vi "Periodic Tasks.vi"(8 "error in":errorcluster) -> ()   [LabVIEW 2017]
doc: "This VI runs in parallel to other tasks. It can contain as many user-defined periodic loops as you need. These can carry out PID or other sorts of timed response."
uses:
  <vilib>/Rock Robotics/WPI/DriverStation/WPI_DriverStationRobotMode2.ctl
  <vilib>/Rock Robotics/WPI/Utilities/WPI_GetSetVariantRefNum.vi
  Robot Global Data.vi
  <vilib>/Rock Robotics/Network Tables/NT Write Number.vi
  <vilib>/Rock Robotics/WPI/ThirdParty/Sensors/ADIS16448 IMU/ADIS16448_IMU.lvlib
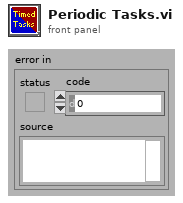
[diagram p1: front panel]
types:
  T1 = typedef "WPI_PotentiometerDevRef.ctl" = cluster{"DevStatus":errorcluster, "Analog Channel":T2, "Invert Output":bool}
  T2 = typedef "FPGA_AIChannel.ctl" = enum8{"AI 0", "AI 1", "AI 2", "AI 3", "AI MXP 0", "AI MXP 1", "AI MXP 2", "AI MXP 3", "Invalid"}
  T3 = typedef "ADIS16448_IMU.lvlib/ADI_IMU_ADIS16448_IMUDevRef.ctl" = cluster{"DevStatus":errorcluster, "Handle":i32, "SPI Bus":T4, "Device Found":bool, "Device Ready":bool, "Yaw Axis":enum16{"X", "Y", "Z"}, "AHRS Algorithm":enum16{"Complementary", "Madgwick"}, "Serial":u16, "Lot ID 2":u16, "Lot ID 1":u16, "Bytes Per Sample":u16, "Calibrate On Open?":bool}
  T4 = typedef "spi_bus.ctl" = enum16{"SPI On-Board, CS0", "SPI On-Board, CS1", "SPI On-Board, CS2", "SPI On-Board, CS3", "SPI MXP", "Invalid"}
  T5 = typedef "WPI_EncoderDevRef.ctl" = cluster{"DevStatus":errorcluster, "EncoderIndex":T6, "CounterIndex":T7, "DistancePerCount":dbl, "Decoding Type":T8}
  T6 = typedef "FPGA_EncoderIdx.ctl" = enum8{"Enc 0", "Enc 1", "Enc 2", "Enc 3", "Enc 4", "Enc 5", "Enc 6", "Enc 7", "Invalid"}
  T7 = typedef "FPGA_CounterCtrSystemIndex.ctl" = enum8{"Ctr 0", "Ctr 1", "Ctr 2", "Ctr 3", "Ctr 4", "Ctr 5", "Ctr 6", "Ctr 7", "Invalid"}
  T8 = typedef "WPI_EncoderType.ctl" = enum16{"1x", "2x", "4x"}
  T9 = typedef "WPI_JoystickDevRef.ctl" = cluster{"Device":T10}
  T10 = typedef "WPI_JoystickDeviceEnum.ctl" = enum16{"USB 0", "USB 1", "USB 2", "USB 3", "USB 4", "USB 5"}
  T11 = typedef "WPI_RobotDriveDevRef.ctl" = cluster{"DevStatus":errorcluster, "Motors[]":T12[], "Square Inputs":bool, "Max Output":dbl}
  T12 = typedef "WPI_MotorControlDeviceRef.ctl" = cluster{"DeviceStatus":errorcluster, "Type":T13, "PWM":cluster{"PWM Channel":T14, "DeadBand":T15}, "CAN":cluster{"Device Number":u8, "SetOutput VI Ref":variant, "GetOutput VI Ref":variant, "Enable VI Ref":variant, "Disable VI Ref":variant, "Data":variant}, "Invert":bool, "DIO PWM":cluster{"PWM \"Enable\" Channel":T14, "DIOChannel":T16, "PWM Rate":dbl}}
  T13 = typedef "WPI_MotorControlType.ctl" = enum16{"PWM", "CAN", "DIO PWM"}
  T14 = typedef "FPGA_DIOPWMChannel.ctl" = enum8{"PWM 0", "PWM 1", "PWM 2", "PWM 3", "PWM 4", "PWM 5", "PWM 6", "PWM 7", "PWM 8", "PWM 9", "PWM MXP 0", "PWM MXP 1", "PWM MXP 2", "PWM MXP 3", "PWM MXP 4", "PWM MXP 5", "PWM MXP 6", "PWM MXP 7", "PWM MXP 8", "PWM MXP 9", "Invalid"}
  T15 = typedef "WPI_PWMDeadband.ctl" = cluster{"Name":string, "maxPositivePwm":i32, "minPositivePwm":i32, "centerPwm":i32, "maxNegativePwm":i32, "minNegativePwm":i32, "angularRange":u16}
  T16 = typedef "FPGA_DIOChannel.ctl" = enum8{"DIO 0", "DIO 1", "DIO 2", "DIO 3", "DIO 4", "DIO 5", "DIO 6", "DIO 7", "DIO 8", "DIO 9", "DIO MXP 0", "DIO MXP 1", "DIO MXP 2", "DIO MXP 3", "DIO MXP 4", "DIO MXP 5", "DIO MXP 6", "DIO MXP 7", "DIO MXP 8", "DIO MXP 9", "DIO MXP 10", "DIO MXP 11", "DIO MXP 12", "DIO MXP 13", "DIO MXP 14", "DIO MXP 15", "SPI Port CS1", "SPI Port CS2", "SPI Port CS3", "SPI Port MISO", "SPI Port MOSI", "Invalid"}
  T17 = cluster{"JoystickDevRef":T9, "RobotDriveDevRef":T11, "PotDevRef":T1, "ADI IMU DevRef":T3, "EncoderDevRef":T5, "EncoderDevRef":T5}
  T18 = typedef "WPI_DriverStationRobotMode2.ctl" = enum16{"Autonomous Disabled", "Autonomous Enabled", "Teleop Disabled", "Teleop Enabled", "Disconnected", "Finish", "Test Disabled", "Test Enabled", "Emergency Stopped"}
  T19 = cluster{"X Angle":dbl, "Y Angle":dbl, "Z Angle":dbl}
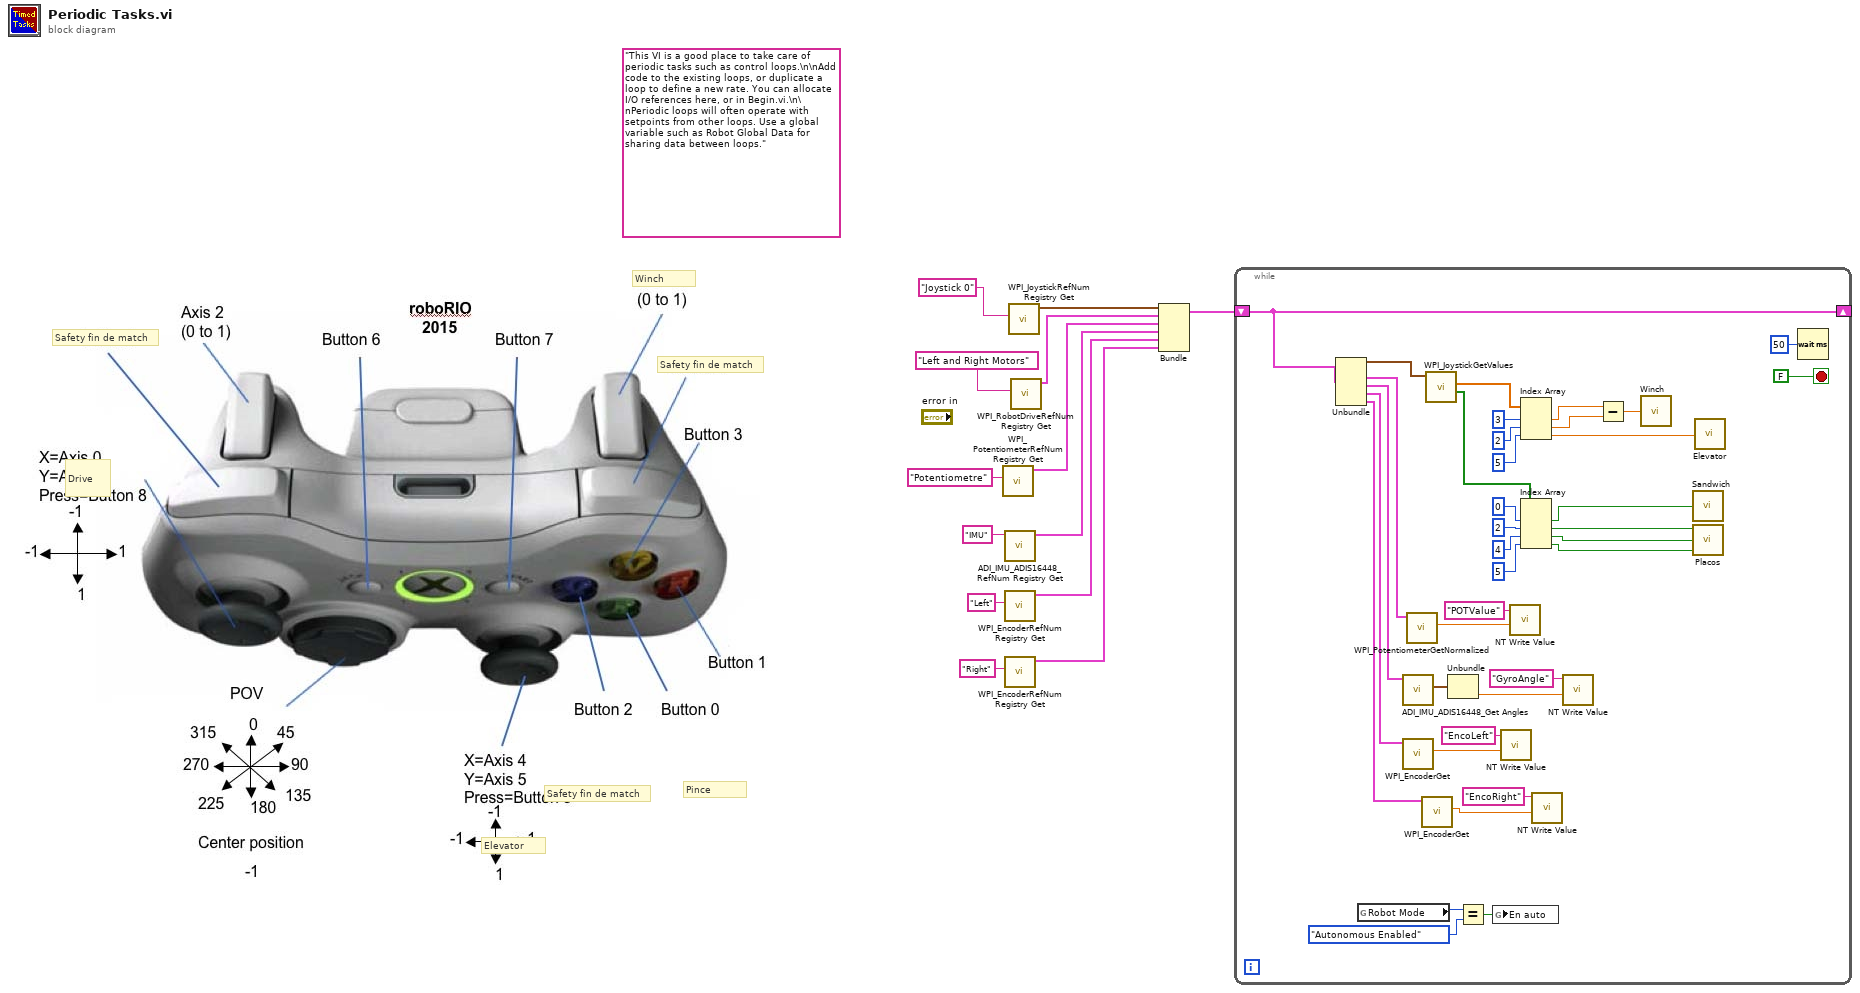
[diagram p0: block diagram]
diagram:
  (unwired) "This VI is a good place to take care of periodic tasks such as control loops.\n\nAdd code to the existing loops, or duplicate a loop to define a new rate. You can allocate I/O references here, or in Begin.vi.\n\nPeriodic loops will often operate with setpoints from other loops. Use a global variable such as Robot Global Data for sharing data between loops."
  # "Safety fin de match"
  # "Safety fin de match"
  # "Safety fin de match"
  # "Pince"
  # "Winch"
  # "Elevator"
  # "Drive"
  n1 = call <vilib>:"WPI_PotentiometerRefNum Registry Get.vi"("refnum name"="Potentiometre") -> ("PotDevRef"=w8:T1)  [unwired: 9 in, 1 out]
  n2 = call <vilib>:"ADI_IMU_ADIS16448_RefNum Registry Get.vi"("refnum name"="IMU") -> ("ADI IMU DevRef"=w7:T3)  [unwired: 9 in, 1 out]
  n3 = call <vilib>:"WPI_EncoderRefNum Registry Get.vi"("refnum name"="Left") -> ("EncoderDevRef"=w2:T5)  [unwired: 9 in, 1 out]
  n4 = call <vilib>:"WPI_EncoderRefNum Registry Get.vi"("refnum name"="Right") -> ("EncoderDevRef"=w1:T5)  [unwired: 9 in, 1 out]
  n5 = call <vilib>:"WPI_JoystickRefNum Registry Get.vi"("refnum name"="Joystick 0") -> ("JoystickDevRef"=w11:T9)  [unwired: 1 in, 9 out]
  n6 = call <vilib>:"WPI_RobotDriveRefNum Registry Get.vi"("refnum name"="Left and Right Motors") -> ("RobotDriveDevRef"=w10:T11)  [unwired: 1 in, 9 out]
  n7 = Bundle("JoystickDevRef"=w11, "RobotDriveDevRef"=w10, "PotDevRef"=w8, "ADI IMU DevRef"=w7, "EncoderDevRef"=w2, "EncoderDevRef"=w1) -> (w9:T17)  [unwired: 1 out]
  n8 = while {
    shift-right: [w48] -> _
    shift-left: w9 -> [w48]
    stop <- FALSE stop-if-true
    n9 = Unbundle(w48) -> ("JoystickDevRef"=w47:T9, "PotDevRef"=w33:T1, "ADI IMU DevRef"=w30:T3, "EncoderDevRef"=w19:T5, "EncoderDevRef"=w18:T5)  [unwired: 1 out]
    n10 = global read "Robot Global Data.vi" "Robot Mode"() -> (w43:T18)
    n11 = call <vilib>:"ADI_IMU_ADIS16448_Get Angles.vi"("ADI IMU DevRef"=w30) -> ("IMU Angles Out"=w29:T19)  [unwired: 7 in, 3 out]
    n12 = call <vilib>:"WPI_EncoderGet.vi"("EncoderDevRef"=w19) -> ("Distance"=w17:dbl)  [unwired: 5 in, 5 out]
    n13 = call <vilib>:"WPI_PotentiometerGetNormalized.vi"("PotDevRef"=w33) -> ("Normalized Value"=w32:dbl)  [unwired: 8 in, 2 out]
    n14 = call <vilib>:"WPI_EncoderGet.vi"("EncoderDevRef"=w18) -> ("Distance"=w16:dbl)  [unwired: 5 in, 5 out]
    n15 = call <vilib>:"WPI_JoystickGetValues.vi"("JoystickDevRef"=w47) -> ("Buttons"=w45:bool[], "Axes"=w46:dbl[])  [unwired: 6 in, 3 out]
    n16 = Unbundle(w29) -> ("Z Angle"=w28:dbl)  [unwired: 2 out]
    n17 = Equal?(x=w43, y=WPI_DriverStationRobotMode2."Autonomous Enabled") -> (x = y?=w41:bool)
    n18 = global write "Robot Global Data.vi" "En auto"(w41) -> ()
    n19 = call-poly <vilib>:"NT Write Value.vi"("Numeric"=w17, "Name"="EncoLeft") -> ()  [unwired: 9 in, 1 out]
    n20 = call-poly <vilib>:"NT Write Value.vi"("Numeric"=w32, "Name"="POTValue") -> ()  [unwired: 9 in, 1 out]
    n21 = Index Array(array=w46, index #1=3 ("index"), index #2=2 ("index"), index #3=5 ("index")) -> (element #1=w36:dbl, element #2=w35:dbl, element #3=w40:dbl)
    n22 = Index Array(array=w45, index #1=0 ("index"), index #2=2 ("index"), index #3=4 ("index"), index #4=5 ("index")) -> (element #1=w44:bool, element #2=w25:bool, element #3=w24:bool, element #4=w23:bool)
    n23 = call-poly <vilib>:"NT Write Value.vi"("Numeric"=w16, "Name"="EncoRight") -> ()  [unwired: 9 in, 1 out]
    n24 = call-poly <vilib>:"NT Write Value.vi"("Numeric"=w28, "Name"="GyroAngle") -> ()  [unwired: 9 in, 1 out]
    n25 = Subtract(x=w36, y=w35) -> (x-y=w34:dbl)
    n26 = call "Winch.vi"("Winch control"=w34) -> ()
    n27 = call "Sandwich.vi"("Pince control teleop"=w44) -> ()
    n28 = call "Placos.vi"("Safety Buttons back 2"=w23, "Safety Buttons back"=w24, "Safety X"=w25) -> ()  [unwired: 2 in]
    n29 = call "Elevator.vi"("Teleop Control"=w40) -> ()
    n30 = Wait (ms)(milliseconds to wait=u32 50) -> ()  [unwired: 1 out]
  }
